vi "open static ref to sequence def interface.vi"(11 "vi name":string) -> (2 "exists":bool, 3 "VI out":refnum<vi>)   [LabVIEW 2018]
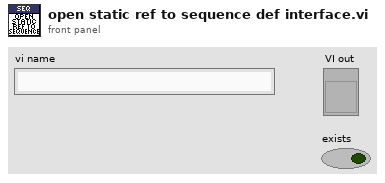
[diagram p1: front panel]
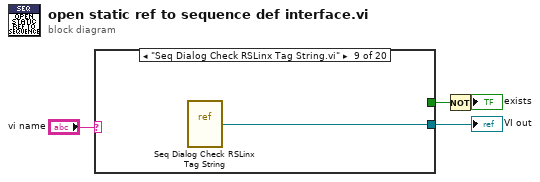
[diagram p0: block diagram]
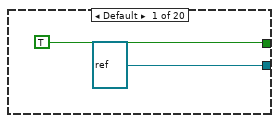
[diagram p2: hidden frame]
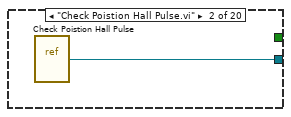
[diagram p3: hidden frame]
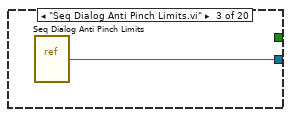
[diagram p4: hidden frame]
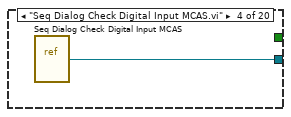
[diagram p5: hidden frame]
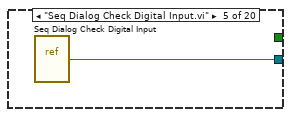
[diagram p6: hidden frame]
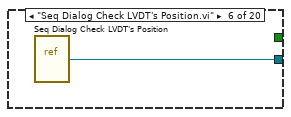
[diagram p7: hidden frame]
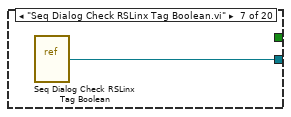
[diagram p8: hidden frame]
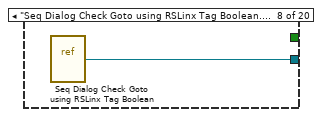
[diagram p9: hidden frame]
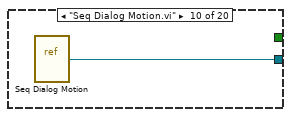
[diagram p10: hidden frame]
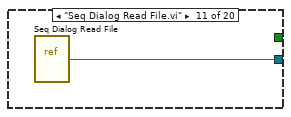
[diagram p11: hidden frame]
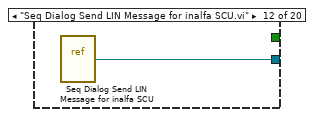
[diagram p12: hidden frame]
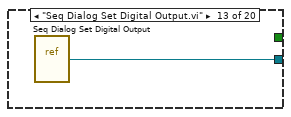
[diagram p13: hidden frame]
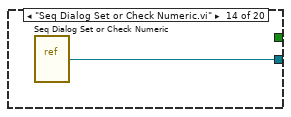
[diagram p14: hidden frame]
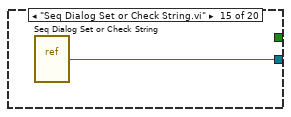
[diagram p15: hidden frame]
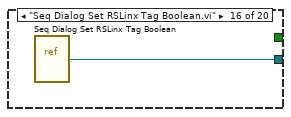
[diagram p16: hidden frame]
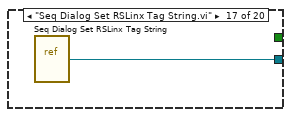
[diagram p17: hidden frame]
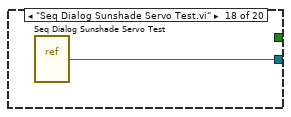
[diagram p18: hidden frame]
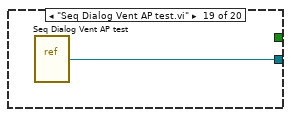
[diagram p19: hidden frame]
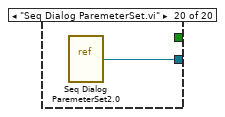
[diagram p20: hidden frame]
diagram:
  n1 = case shown="\"Seq Dialog Check RSLinx Tag String.vi\"" "vi name" {
    tunnel: [TRUE _ _ _ _ _ _ _ _ _ _ _ _ _ _ _ _ _ _ _] -> w2
    tunnel: [refnum<vi> refnum w7 w8 w9 w10 w11 w12 w13 w14 w15 w16 w17 w18 w19 w20 w21 w22 w23 w24 w25] -> w4
    frame Default {
    }
    frame "Check Poistion Hall Pulse.vi" {
      n2 = vi-ref "Check Poistion Hall Pulse.vi"() -> (w7:refnum<vi>)
    }
    frame "Seq Dialog Anti Pinch Limits.vi" {
      n3 = vi-ref "Seq Dialog Anti Pinch Limits.vi"() -> (w8:refnum<vi>)
    }
    frame "Seq Dialog Check Digital Input MCAS.vi" {
      n4 = vi-ref "Seq Dialog Check Digital Input MCAS.vi"() -> (w9:refnum<vi>)
    }
    frame "Seq Dialog Check Digital Input.vi" {
      n5 = vi-ref "Seq Dialog Check Digital Input.vi"() -> (w10:refnum<vi>)
    }
    frame "Seq Dialog Check LVDT's Position.vi" {
      n6 = vi-ref "Seq Dialog Check LVDT's Position.vi"() -> (w11:refnum<vi>)
    }
    frame "Seq Dialog Check RSLinx Tag Boolean.vi" {
      n7 = vi-ref "Seq Dialog Check RSLinx Tag Boolean.vi"() -> (w12:refnum<vi>)
    }
    frame "Seq Dialog Check Goto using RSLinx Tag Boolean.vi" {
      n8 = vi-ref "Seq Dialog Check Goto using RSLinx Tag Boolean.vi"() -> (w13:refnum<vi>)
    }
    frame "Seq Dialog Check RSLinx Tag String.vi" {
      n9 = vi-ref "Seq Dialog Check RSLinx Tag String.vi"() -> (w14:refnum<vi>)
    }
    frame "Seq Dialog Motion.vi" {
      n10 = vi-ref "Seq Dialog Motion.vi"() -> (w15:refnum<vi>)
    }
    frame "Seq Dialog Read File.vi" {
      n11 = vi-ref "Seq Dialog Read File.vi"() -> (w16:refnum<vi>)
    }
    frame "Seq Dialog Send LIN Message for inalfa SCU.vi" {
      n12 = vi-ref "Seq Dialog Send LIN Message for inalfa SCU.vi"() -> (w17:refnum<vi>)
    }
    frame "Seq Dialog Set Digital Output.vi" {
      n13 = vi-ref "Seq Dialog Set Digital Output.vi"() -> (w18:refnum<vi>)
    }
    frame "Seq Dialog Set or Check Numeric.vi" {
      n14 = vi-ref "Seq Dialog Set or Check Numeric.vi"() -> (w19:refnum<vi>)
    }
    frame "Seq Dialog Set or Check String.vi" {
      n15 = vi-ref "Seq Dialog Set or Check String.vi"() -> (w20:refnum<vi>)
    }
    frame "Seq Dialog Set RSLinx Tag Boolean.vi" {
      n16 = vi-ref "Seq Dialog Set RSLinx Tag Boolean.vi"() -> (w21:refnum<vi>)
    }
    frame "Seq Dialog Set RSLinx Tag String.vi" {
      n17 = vi-ref "Seq Dialog Set RSLinx Tag String.vi"() -> (w22:refnum<vi>)
    }
    frame "Seq Dialog Sunshade Servo Test.vi" {
      n18 = vi-ref "Seq Dialog Sunshade Servo Test.vi"() -> (w23:refnum<vi>)
    }
    frame "Seq Dialog Vent AP test.vi" {
      n19 = vi-ref "Seq Dialog Vent AP test.vi"() -> (w24:refnum<vi>)
    }
    frame "Seq Dialog ParemeterSet.vi" {
      n20 = vi-ref "Seq Dialog ParemeterSet2.0.vi"() -> (w25:refnum<vi>)
    }
  }
  "VI out" <- w4
  n21 = Not(x=w2) -> (.not. x?=→"exists":bool)
